vi "Init.vi"(8 "error in (no error)":errorcluster, 11 "MultiPlotPanel in":refnum<class "MultiPlotPanel.lvclass">) -> (0 "error out":errorcluster, 2 "RocketPlotPanel Type":refnum<class "RocketPlotPanel.lvclass">, 3 "MultiPlotPanel out":refnum<class "MultiPlotPanel.lvclass">)   [LabVIEW 2021, in "MultiStokePlot.lvlib" / "MultiPlotPanel.lvclass"]
uses:
  MultiPlotPanel.lvclass
  <userlib>/bjustice/RocketPlot/Classes/RocketPlotPanel/RocketPlotPanel.lvclass
  MultiPlotPanel.lvclass/MultiPlotPanel.ctl
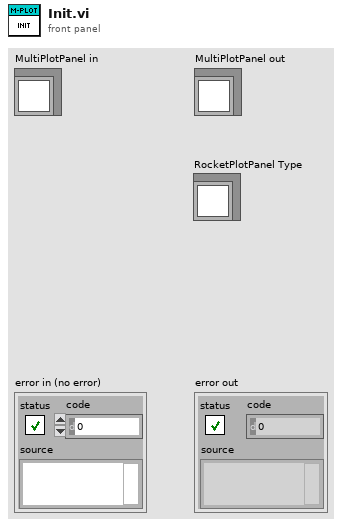
[diagram p1: front panel]
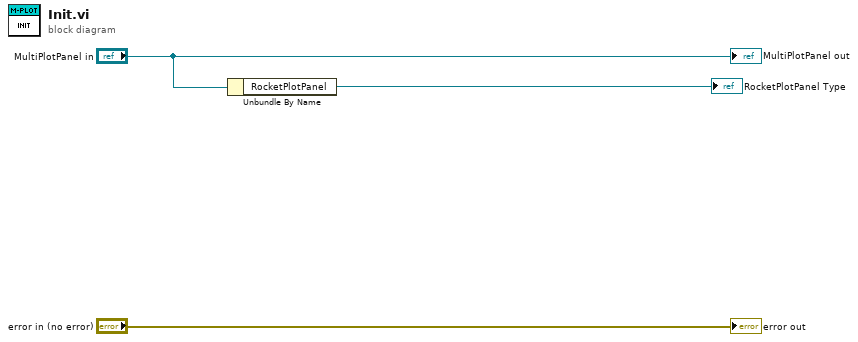
[diagram p0: block diagram]
diagram:
  n1 = Unbundle By Name("MultiPlotPanel in") -> ("RocketPlotPanel"=→"RocketPlotPanel Type":refnum<class "RocketPlotPanel.lvclass">)
  "error out" <- "error in (no error)"
  "MultiPlotPanel out" <- "MultiPlotPanel in"
